vi "read system session.vi"(8 "error in":errorcluster, 11 "syscfg device in":refnum<class "SysCfg Device.lvclass">) -> (0 "error out":errorcluster, 2 "system session":refnum<data-value>, 3 "syscfg device out":refnum<class "SysCfg Device.lvclass">)   [LabVIEW 2013, in "SMI.lvlib" / "SysCfg Device.lvclass"]
uses:
  SysCfg Device.lvclass
  SysCfg Device.lvclass/SysCfg Device.ctl
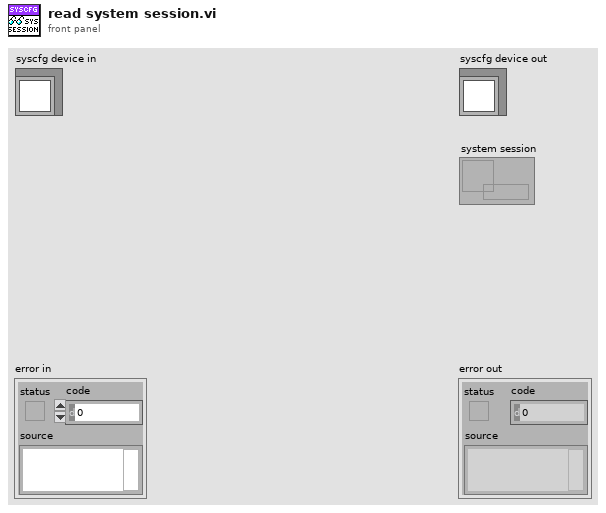
[diagram p1: front panel]
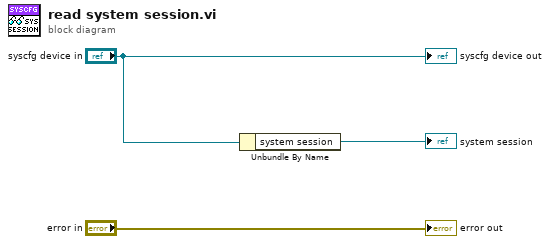
[diagram p0: block diagram]
diagram:
  n1 = Unbundle By Name("syscfg device in") -> ("system session"=→"system session":refnum<data-value>)
  "error out" <- "error in"
  "syscfg device out" <- "syscfg device in"
